vi "Get Target Properties.vi"(8 "error in":errorcluster, 11 "target ref in":refnum<k24>) -> (0 "error out":errorcluster, 1 "TL timeout value":dbl=120.0 format="%#_13g", 2 "ts value":u32, 3 "target ref out":refnum<k24>, 4 "dependent node found":bool, 5 "dependent custom device node path":string)   [LabVIEW 2026]
uses:
  NationalInstruments.VeriStand.SystemStorage
  NationalInstruments.VeriStand.SystemDefinitionAPI
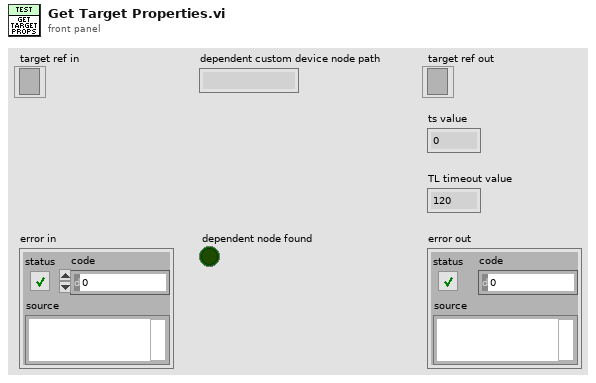
[diagram p1: front panel]
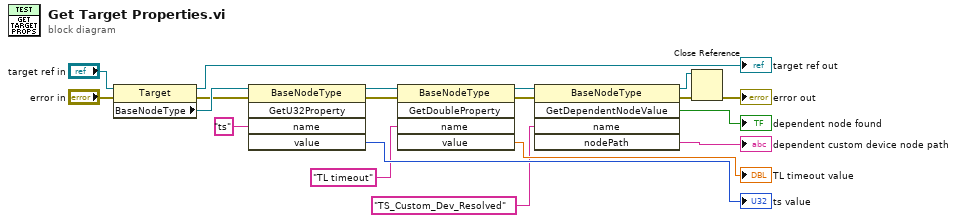
[diagram p0: block diagram]
diagram:
  n1 = property class="Target"(reference="target ref in", error in="error in") -> (reference out=→"target ref out":refnum<k24>, error out=w2:errorcluster, "BaseNodeType"=w18:refnum<k24>)
  n2 = invoke class="BaseNodeType" method="GetU32Property"(reference=w18, error in=w2, "name"="ts") -> (reference out=w14:refnum<k24>, error out=w15:errorcluster, "value"=→"ts value":u32)  [unwired: 2 in, 2 out]
  n3 = invoke class="BaseNodeType" method="GetDoubleProperty"(reference=w14, error in=w15, "name"="TL timeout") -> (reference out=w7:refnum<k24>, error out=w8:errorcluster, "value"=→"TL timeout value":dbl)  [unwired: 2 in, 2 out]
  n4 = invoke class="BaseNodeType" method="GetDependentNodeValue"(reference=w7, error in=w8, "name"="TS_Custom_Dev_Resolved") -> (reference out=w5:refnum<k24>, error out=w6:errorcluster, "GetDependentNodeValue"=→"dependent node found":bool, "nodePath"=→"dependent custom device node path":string)  [unwired: 2 in, 1 out]
  n5 = Close Reference(reference=w5, error in (no error)=w6) -> (error out=→"error out":errorcluster)
